vi "Read from Hardware.vi"(8 "error in":errorcluster, 10 "values in":dbl[](array[numeric]), 11 "logging execution unit":refnum<class "Logging Execution Unit.lvclass">) -> (0 "error out":errorcluster, 2 "values out":dbl[](array[numeric]), 3 "logging execution unit out":refnum<class "Logging Execution Unit.lvclass">)   [LabVIEW 2020, in "AIM MIL-STD-1553 Engine.lvlib" / "Implementation.lvlib" / "Logging Execution Unit.lvclass"]
uses:
  Logging Execution Unit.lvclass
  C:/dev/git/niveristand-aim-milStd1553-custom-device/Source/Custom Device Support/Engine/Implementation/Execution Unit/Execution Unit.lvclass
  Execution Unit/Execution Unit.lvclass/Execution Unit.ctl
  Logging Execution Unit.lvclass/Logging Execution Unit.ctl
  Hardware API/AIM MIL-STD-1553 Hardware API.lvlib
  Execution Unit/Execution Unit.lvclass
  Logging/Word Logging/Word Logging.lvlib
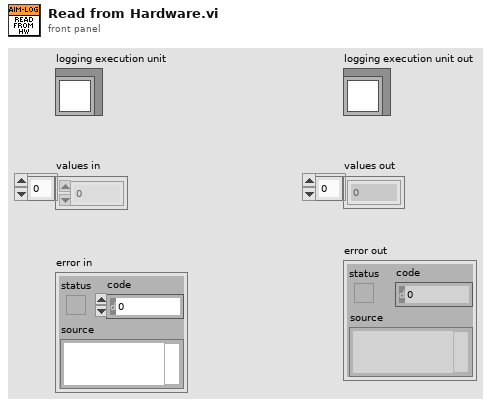
[diagram p1: front panel]
types:
  T1 = typedef "AIM MIL-STD-1553 Hardware API.lvlib/Module Reference.ctl" = u32
  T2 = typedef "Log Entry.ctl" = cluster{"Queue Entry":T3, "Message Data Buffer":u16[]}
  T3 = typedef "1553 BM Queue Entry.ctl" = cluster{"RT Address":u8, "Sub-address":u8, "Mode Code":enum16{"Dynamic bus control", "Synchronize", "Transmit status word", "Initiate self test", "Transmitter shutdown", "Override transmitter shutdown", "Inhibit terminal flag bit", "Override inhibit terminal flag bit", "Reset remote terminal", "(reserved)", "(reserved) ", "(reserved)  ", "(reserved)   ", "(reserved)    ", "(reserved)     ", "(reserved)      ", "Transmit vector word", "Synchronize ", "Transmit last command", "Transmit bit word", "Selected xmtr shutdown", "Override selected xmtr shutdown", "(reserved)       ", "(reserved)        ", "(reserved)         ", "(reserved)          ", "(reserved)           ", "(reserved)            ", "(reserved)             ", "(reserved)              ", "(reserved)               ", "(reserved)                "}, "Direction":enum16{"receive", "transmit"}, "Type":enum16{"sub-address", "mode code"}, "RT Address 2":u8, "Sub-address 2":u8, "Mode Code 2":enum16{"Dynamic bus control", "Synchronize", "Transmit status word", "Initiate self test", "Transmitter shutdown", "Override transmitter shutdown", "Inhibit terminal flag bit", "Override inhibit terminal flag bit", "Reset remote terminal", "(reserved)", "(reserved) ", "(reserved)  ", "(reserved)   ", "(reserved)    ", "(reserved)     ", "(reserved)      ", "Transmit vector word", "Synchronize ", "Transmit last command", "Transmit bit word", "Selected xmtr shutdown", "Override selected xmtr shutdown", "(reserved)       ", "(reserved)        ", "(reserved)         ", "(reserved)          ", "(reserved)           ", "(reserved)            ", "(reserved)             ", "(reserved)              ", "(reserved)               ", "(reserved)                "}, "Direction 2":enum16{"receive", "transmit"}, "Type 2":enum16{"sub-address", "mode code"}, "Word Count":u8, "Bus":enum16{"primary", "secondary"}, "Minutes":i32, "Seconds":i32, "Microseconds":i32, "Error ":enum16{"No error", "Terminal no response error", "Manchester coding error", "High bit count error", "Low bit count error", "Parity error", "Inverted sync error", "Interw ord gap error", "Transmission on both MILbus channels", "Reserved mode code error", "Early response or gap too short", "ME bit set in status word", "Status word exception error", "High wordcount error", "Low wordcount error", "Illegal command word"}}
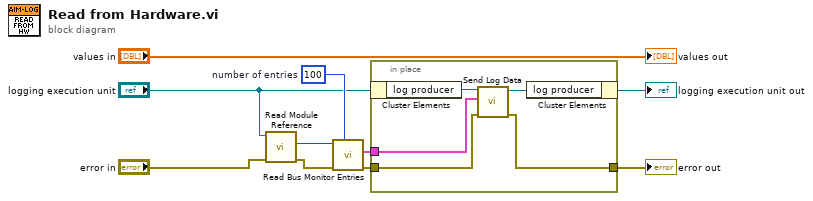
[diagram p0: block diagram]
diagram:
  w8 = 100  # number of entries
  n1 = call "Read Module Reference.vi"("error in"="error in", "execution unit"="logging execution unit") -> ("error out"=w6:errorcluster, "module reference"=w7:T1)  [unwired: 7 in, 1 out]
  n2 = call "Read Bus Monitor Entries.vi"("number of entries"=w8, "error in"=w6, "module handle"=w7) -> ("error out"=w2:errorcluster, "Array"=w1:T2[])  [unwired: 6 in, 1 out]
  n3 = in-place {
    in-place-border: [w12] -> w3
    in-place-border: w2 -> [w13]
    in-place-border: w1 -> [w11]
    n4 = in-place-cluster #1("logging execution unit") -> ("log producer"=w15:refnum<class "Log Producer.lvclass">)
    n5 = call "Send Log Data.vi"("error in"=w13, "Data"=w11, "Producer in"=w15) -> ("error out"=w12:errorcluster, "Producer out"=w14:refnum<class "Log Producer.lvclass">)  [unwired: 7 in]
    n6 = in-place-cluster #1("log producer"=w14) -> (→"logging execution unit out":refnum<class "Logging Execution Unit.lvclass">)
  }
  "error out" <- w3
  "values out" <- "values in"
